vi "Trace Engine.vi"(0 "FPGA VI Reference":refnum<k20>, 7 "Arr Refnum":refnum<vi>, 11 "TraceCluster":refnum<vi>) -> ()   [LabVIEW 2013]
uses:
  <vilib>/rvi/interface/nirviMethod/nirviMethod.xnode
  <vilib>/FPGAPlugInAG/Dynamic/niLvFpga_ReadFifo_Dynamic.vi
  <vilib>/rvi/errors/niLvFpgaMergeErrorWithErrorCode.vi
  Controls/TraceCluster.ctl
  <vilib>/ptbypt/NI_PtbyPt.lvlib
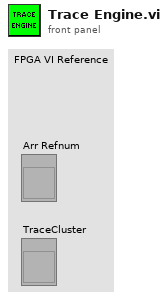
[diagram p1: front panel]
types:
  T1 = typedef "TraceCluster.ctl" = cluster{"PreTriggerPts":i32, "TotalPts":i32, "TriggerLvl":dbl, "PlotStyle":enum16{"Single - Rising Edge", "Single - Falling Edge", "Continuous", "Repeat - Rising Edge", "Repeat - Falling Edge"}, "TriggerChannel":i32, "TraceCtrl":bool}
  T2 = cluster{"rt fifo":refnum<k33>, "FPGA VI Reference":refnum<k20>, "Stored Data":dbl[][], "TraceCluster":T1, "TraceClusterRef":refnum<vi>, "InSync":bool, "Cal Array":dbl[][]}
  T3 = enum16{"Single - Rising Edge", "Single - Falling Edge", "Continuous", "Repeat - Rising Edge", "Repeat - Falling Edge"}
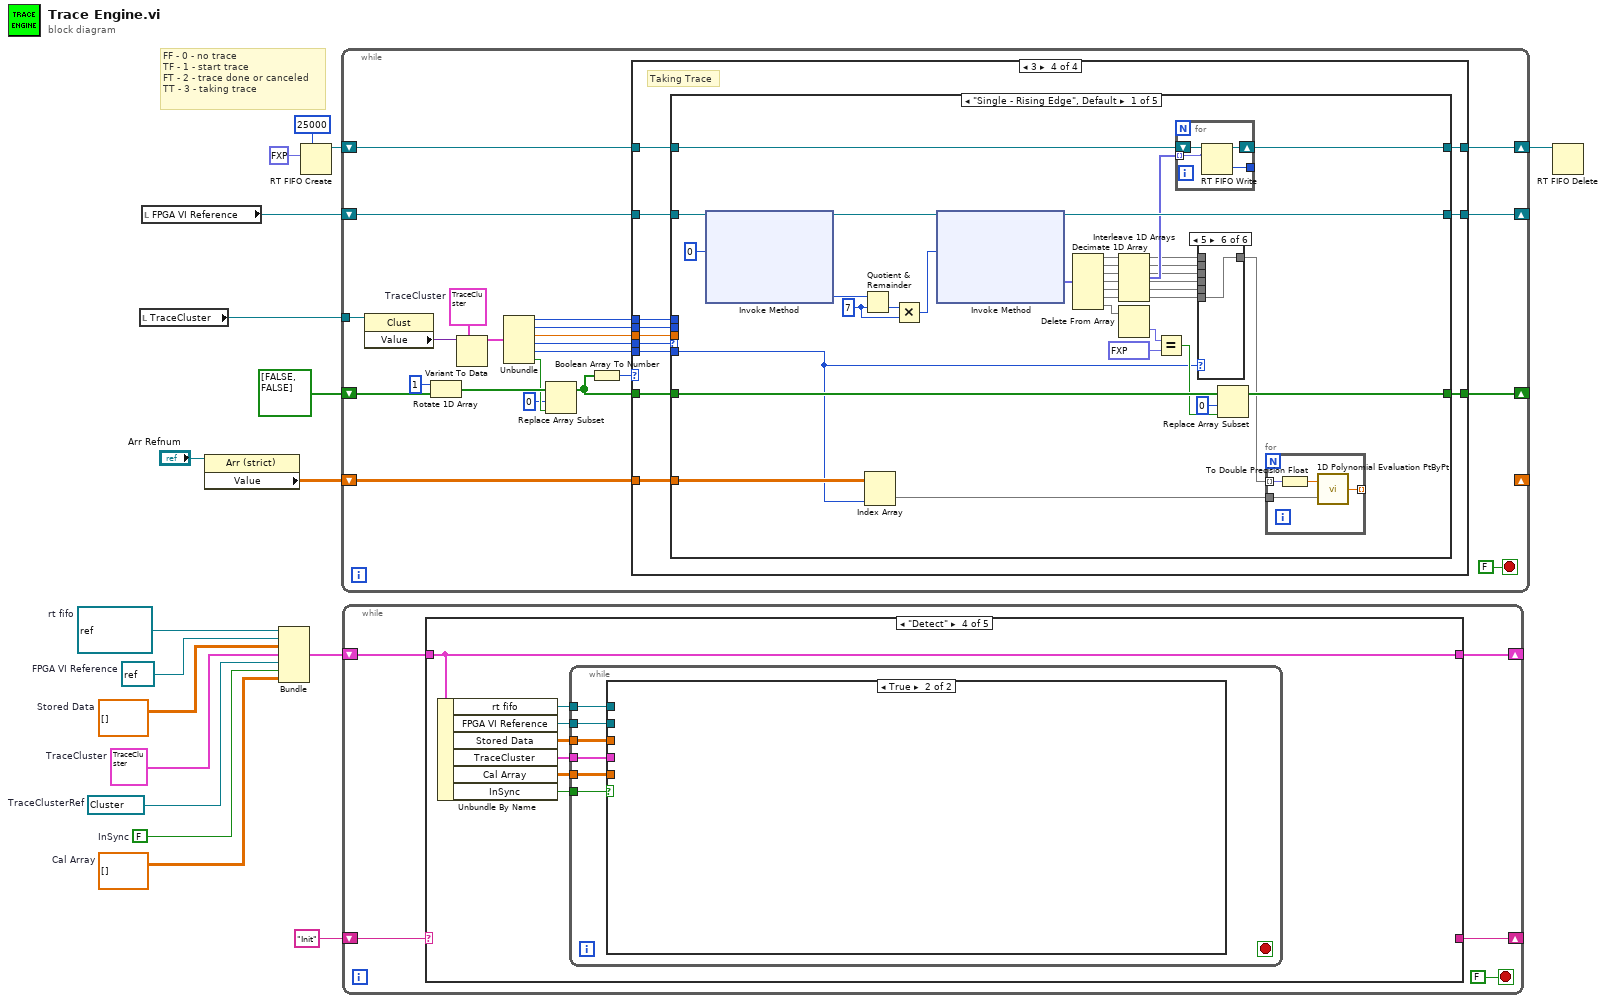
[diagram p0: block diagram]
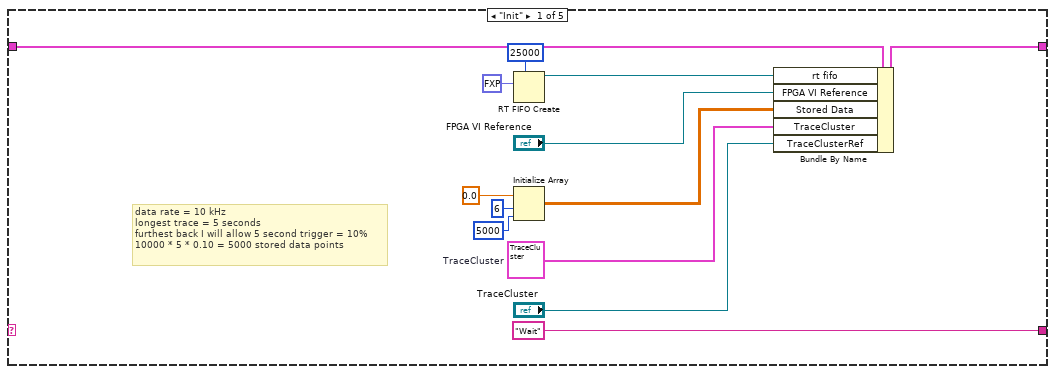
[diagram p2: hidden frame]
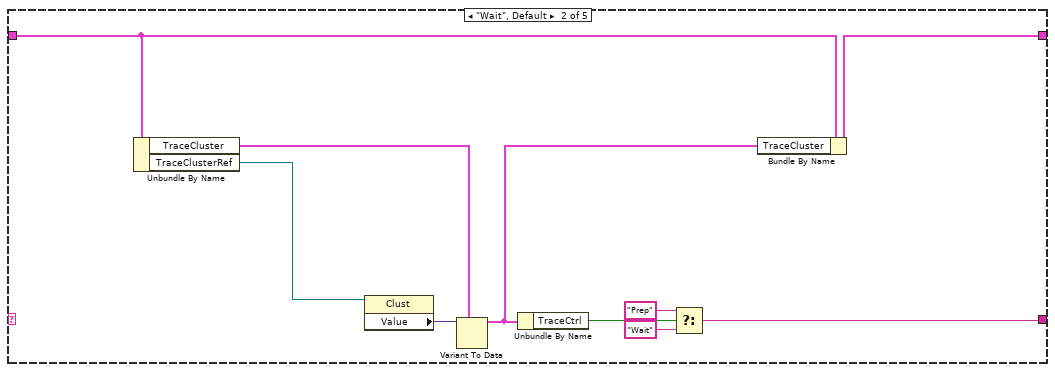
[diagram p3: hidden frame]
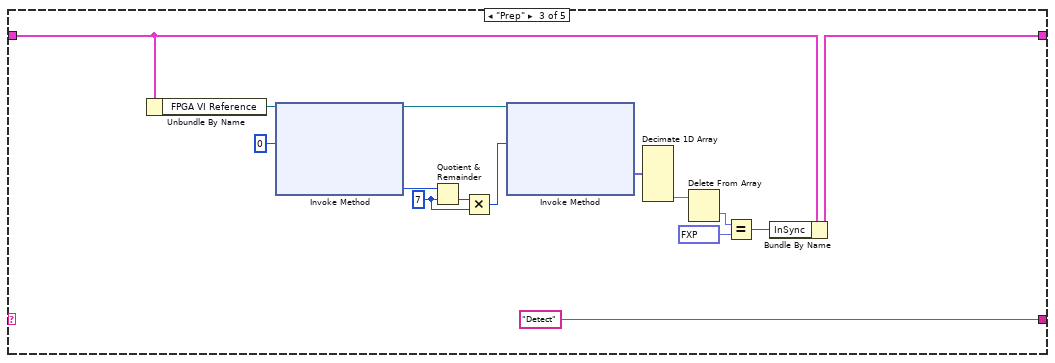
[diagram p4: hidden frame]
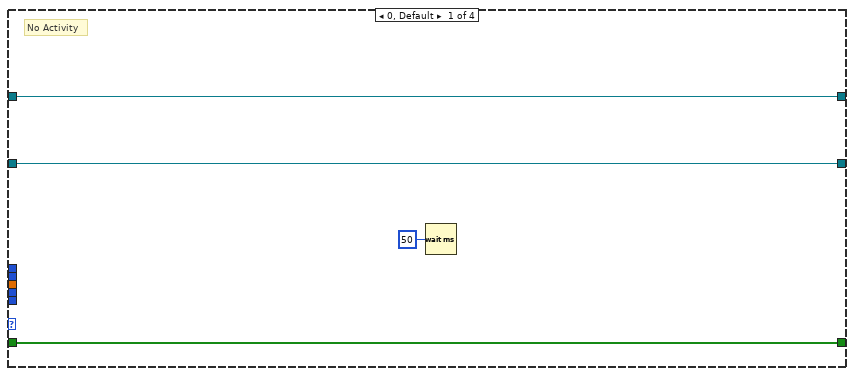
[diagram p7: hidden frame]
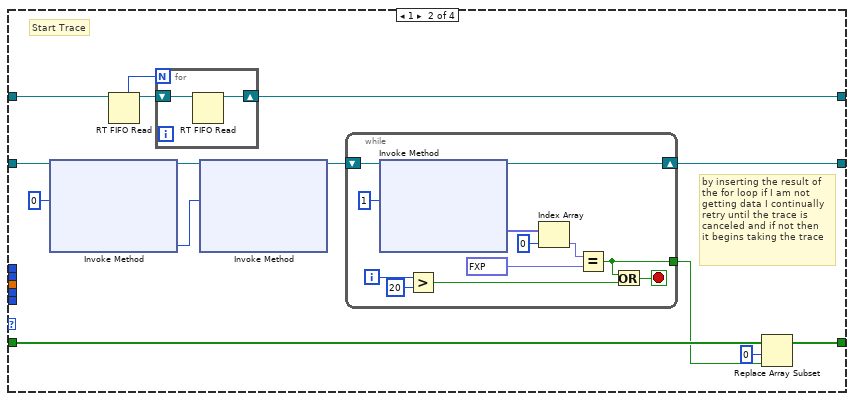
[diagram p8: hidden frame]
diagram:
  w1 = dbl[][] []  # Cal Array
  w3 = FALSE  # InSync
  w4 = refnum<vi> refnum  # TraceClusterRef
  w5 = T1 {"PreTriggerPts"=0, "TotalPts"=0, "TriggerLvl"=0.0, "PlotStyle"=enum."Single - Rising Edge", "TriggerChannel"=0, "TraceCtrl"=FALSE}  # TraceCluster
  w6 = dbl[][] []  # Stored Data
  w7 = refnum<k20> refnum  # FPGA VI Reference
  w8 = refnum<k33> refnum  # rt fifo
  # "FF - 0 - no trace\nTF - 1 - start trace\nFT - 2 - trace done or canceled\nTT - 3 - taking trace"
  n1 = local read "TraceCluster"() -> (w9:refnum<vi>)
  n2 = local read "FPGA VI Reference"() -> (w10:refnum<k20>)
  n3 = property class="Arr (strict)"(reference="Arr Refnum") -> ("Value"=w12:dbl[][])  [unwired: 1 in, 2 out]
  n4 = Bundle("rt fifo"=w8, "FPGA VI Reference"=w7, "Stored Data"=w6, "TraceCluster"=w5, "TraceClusterRef"=w4, "InSync"=w3, "Cal Array"=w1) -> (w2:T2)  [unwired: 1 in]
  n5 = RT FIFO Create(1:fxp<+/-,25,15> 0.0, 4:u32 25000 ("size (10)")) -> (8:w16:refnum<k33>)  [unwired: 6 in, 2 out]
  n6 = while {
    tunnel: w9 -> [w33]
    shift-right: [w22] -> _
    shift-left: bool[] [FALSE, FALSE] -> [w31]
    shift-right: [w24] -> _
    shift-left: w10 -> [w25]
    shift-right: [w20] -> w15
    shift-left: w16 -> [w21]
    shift-right: _ -> [_]
    shift-left: w12 -> [w19]
    stop <- FALSE stop-if-true
    w35 = T1 {"PreTriggerPts"=0, "TotalPts"=0, "TriggerLvl"=0.0, "PlotStyle"=enum."Single - Rising Edge", "TriggerChannel"=0, "TraceCtrl"=FALSE}  # TraceCluster
    n7 = property class="Clust"(reference=w33) -> ("Value"=w34:variant)  [unwired: 1 in, 2 out]
    n8 = Rotate 1D Array(1:w31, 2:1 ("n")) -> (0:w29:bool[])
    n9 = Variant To Data(type=w35, Variant=w34) -> (data=w32:T1)  [unwired: 1 in, 1 out]
    n10 = Unbundle(w32) -> ("PreTriggerPts"=w36:i32, "TotalPts"=w37:i32, "TriggerLvl"=w38:dbl, "PlotStyle"=w40:T3, "TriggerChannel"=w39:i32, "TraceCtrl"=w28:bool)
    n11 = Replace Array Subset(array=w29, new element=w28, index=0) -> (w23:bool[])
    n12 = Boolean Array To Number(Boolean array=w23) -> (number=w26:u32)
    n13 = case shown="3" w26 {
      tunnel: w25 -> [w44 w59 w76 w88]
      tunnel: w40 -> [_ _ _ w84]
      tunnel: w39 -> [_ _ _ w83]
      tunnel: w38 -> [_ _ _ w85]
      tunnel: w37 -> [_ _ _ w86]
      tunnel: w36 -> [_ _ _ w87]
      tunnel: [w44 w54 w76 w80] -> w24
      tunnel: w23 -> [w43 w53 w75 w79]
      tunnel: [w43 w52 w75 w78] -> w22
      tunnel: w21 -> [w42 w49 w74 w82]
      tunnel: [w42 w46 w74 w81] -> w20
      tunnel: w19 -> [_ _ _ w77]
      frame 0, Default {
        # "No Activity"
        n14 = Wait (ms)(milliseconds to wait=u32 50) -> ()  [unwired: 1 out]
      }
      frame 1 {
        # "Start Trace"
        # "by inserting the result of\nthe for loop if I am not\ngetting data I continually\nretry until the trace is\ncanceled and if not then\nit begins taking the trace"
        n15 = xnode "Invoke Method"("FPGA VI Reference In"=w59, "Number of Elements"=u32 0) -> ("FPGA VI Reference Out"=w58:refnum<k20>, "Elements Remaining"=w55:u32)  [unwired: 2 in, 2 out]
        n16 = RT FIFO Read(0:w49) -> (7:w47:u32, 8:w48:refnum<k33>)  [unwired: 3 in, 3 out]
        n17 = for {
          N: w47 -> [_]
          shift-right: [w60] -> w46
          shift-left: w48 -> [w61]
          n18 = RT FIFO Read(0:w61) -> (8:w60:refnum<k33>)  [unwired: 3 in, 4 out]
        }
        n19 = xnode "Invoke Method"("FPGA VI Reference In"=w58, "Number of Elements"=w55) -> ("FPGA VI Reference Out"=w57:refnum<k20>)  [unwired: 2 in, 3 out]
        n20 = while {
          shift-right: [w64] -> w54
          shift-left: w57 -> [w72]
          tunnel: [w62] -> w50
          i -> [w67]
          stop <- w65 stop-if-true
          n21 = xnode "Invoke Method"("FPGA VI Reference In"=w72, "Number of Elements"=u32 1) -> ("FPGA VI Reference Out"=w64:refnum<k20>, "Data"=w70:fxp<+/-,25,15>[])  [unwired: 2 in, 2 out]
          n22 = Greater?(x=w67, y=20) -> (0:w63:bool)
          n23 = Index Array(array=w70, index=0) -> (element=w68:fxp<+/-,25,15>)
          n24 = Equal?(x=w68, y=fxp<+/-,1,15> -16384.0) -> (x = y?=w62:bool)
          n25 = Or(x=w62, y=w63) -> (x .or. y?=w65:bool)
        }
        n26 = Replace Array Subset(array=w53, new element=w50, index=0) -> (w52:bool[])
      }
      frame 2 {
        # "Trace Canceled OR Trace Complete"
      }
      frame 3 {
        # "Taking Trace"
        n27 = case shown="\"Single - Rising Edge\", Default" w84 {
          tunnel: w83 -> [w96 _ _ _ _]
          tunnel: w85 -> [_ _ _ _ _]
          tunnel: w86 -> [_ _ _ _ _]
          tunnel: w87 -> [_ _ _ _ _]
          tunnel: w88 -> [w116 _ _ _ _]
          tunnel: w82 -> [w114 _ _ _ _]
          tunnel: [w109 _ _ _ _] -> w81
          tunnel: [w108 _ _ _ _] -> w80
          tunnel: w79 -> [w104 _ _ _ _]
          tunnel: [w103 _ _ _ _] -> w78
          tunnel: w77 -> [w98 _ _ _ _]
          frame "Single - Rising Edge", Default {
            w111 = u32 7 ("y")
            n28 = xnode "Invoke Method"("FPGA VI Reference In"=w116, "Number of Elements"=u32 0) -> ("FPGA VI Reference Out"=w115:refnum<k20>, "Elements Remaining"=w113:u32)  [unwired: 2 in, 2 out]
            n29 = Quotient & Remainder(x=w113, y=w111) -> (floor(x/y)=w112:u32)  [unwired: 1 out]
            n30 = Index Array(array=w98, index (col)=w96) -> (element=w97:dbl[])  [unwired: 1 in]
            n31 = Multiply(x=w112, y=w111) -> (x*y=w110:u32)
            n32 = xnode "Invoke Method"("FPGA VI Reference In"=w115, "Number of Elements"=w110) -> ("FPGA VI Reference Out"=w108:refnum<k20>, "Data"=w107:fxp<+/-,25,15>[])  [unwired: 2 in, 2 out]
            n33 = Decimate 1D Array(w107) -> (w95:fxp<+/-,25,15>[], w94:fxp<+/-,25,15>[], w93:fxp<+/-,25,15>[], w92:fxp<+/-,25,15>[], w91:fxp<+/-,25,15>[], w90:fxp<+/-,25,15>[], w100:fxp<+/-,25,15>[])
            n34 = Interleave 1D Arrays(w95, w94, w93, w92, w91, w90) -> (w99:fxp<+/-,25,15>[])
            n35 = Delete From Array(array=w100) -> (deleted portion=w106:fxp<+/-,25,15>)  [unwired: 2 in, 1 out]
            n36 = Equal?(x=w106, y=fxp<+/-,25,15> -16384.0) -> (x = y?=w102:bool)
            n37 = for {
              tunnel: [w128] -> _ mode=indexing
              shift-right: [w130] -> w109
              shift-left: w114 -> [w131]
              tunnel: [w129] -> _
              tunnel: w99 -> [w128] mode=indexing
              n38 = RT FIFO Write(0:w131, 1:w128) -> (7:w129:u32, 8:w130:refnum<k33>)  [unwired: 3 in, 2 out]
            }
            n39 = case shown="5" w96 {
              tunnel: w95 -> [w118 _ _ _ _ _]
              tunnel: w94 -> [_ w119 _ _ _ _]
              tunnel: w93 -> [_ _ w120 _ _ _]
              tunnel: w92 -> [_ _ _ w121 _ _]
              tunnel: w91 -> [_ _ _ _ w122 _]
              tunnel: w90 -> [_ _ _ _ _ w123]
              tunnel: [w118 w119 w120 w121 w122 w123] -> w89
              frame 0, Default {
              }
              frame 1 {
              }
              frame 2 {
              }
              frame 3 {
              }
              frame 4 {
              }
              frame 5 {
              }
            }
            n40 = Replace Array Subset(array=w104, new element=w102, index=0) -> (w103:bool[])
            n41 = for {
              tunnel: w97 -> [w127]
              tunnel: w89 -> [w125] mode=indexing
              tunnel: [w126] -> _ mode=indexing
              n42 = To Double Precision Float(number=w125) -> (double precision float=w124:dbl)
              n43 = call <vilib>:"1D Polynomial Evaluation PtByPt.vi"("Coefficients: a"=w127, "x"=w124) -> ("y"=w126:dbl)
            }
          }
          frame "Single - Falling Edge" {
          }
          frame "Continuous" {
          }
          frame "Repeat - Rising Edge" {
          }
          frame "Repeat - Falling Edge" {
          }
        }
      }
    }
  }
  n44 = while {
    shift-right: [w134] -> _
    shift-left: "Init" -> [w135]
    shift-right: [w132] -> _
    shift-left: w2 -> [w133]
    stop <- FALSE stop-if-true
    n45 = case shown="\"Detect\"" w135 {
      tunnel: ["Wait" w155 "Detect" _ _] -> w134
      tunnel: w133 -> [w143 w152 w162 w181 _]
      tunnel: [w137 w151 w161 w181 _] -> w132
      frame "Init" {
        w139 = T1 {"PreTriggerPts"=0, "TotalPts"=0, "TriggerLvl"=0.0, "PlotStyle"=enum."Single - Rising Edge", "TriggerChannel"=0, "TraceCtrl"=FALSE}  # TraceCluster
        # "data rate = 10 kHz\nlongest trace = 5 seconds\nfurthest back I will allow 5 second trigger = 10%\n10000 * 5 * 0.10 = 5000 stored data points"
        n46 = RT FIFO Create(1:fxp<+/-,25,15> 0.0, 4:u32 25000 ("size (10)")) -> (8:w142:refnum<k33>)  [unwired: 6 in, 2 out]
        n47 = Initialize Array(0.0 ("element"), 6 ("dimension size"), 5000 ("dimension size")) -> (w140:dbl[][])
        n48 = Bundle By Name(cluster=w143, "rt fifo"=w142, "FPGA VI Reference"="FPGA VI Reference", "Stored Data"=w140, "TraceCluster"=w139, "TraceClusterRef"="TraceCluster") -> (w137:T2)
      }
      frame "Wait", Default {
        n49 = Unbundle By Name(w152) -> ("TraceCluster"=w153:T1, "TraceClusterRef"=w154:refnum<vi>)
        n50 = property class="Clust"(reference=w154) -> ("Value"=w159:variant)  [unwired: 1 in, 2 out]
        n51 = Variant To Data(type=w153, Variant=w159) -> (data=w150:T1)  [unwired: 1 in, 1 out]
        n52 = Unbundle By Name(w150) -> ("TraceCtrl"=w158:bool)
        n53 = Select(t="Prep", s=w158, f="Wait") -> (s? t:f=w155:string)
        n54 = Bundle By Name(cluster=w152, "TraceCluster"=w150) -> (w151:T2)
      }
      frame "Prep" {
        w168 = u32 7 ("y")
        n55 = Unbundle By Name(w162) -> ("FPGA VI Reference"=w164:refnum<k20>)
        n56 = xnode "Invoke Method"("FPGA VI Reference In"=w164, "Number of Elements"=u32 0) -> ("FPGA VI Reference Out"=w163:refnum<k20>, "Elements Remaining"=w166:u32)  [unwired: 2 in, 2 out]
        n57 = Quotient & Remainder(x=w166, y=w168) -> (floor(x/y)=w167:u32)  [unwired: 1 out]
        n58 = Multiply(x=w167, y=w168) -> (x*y=w169:u32)
        n59 = xnode "Invoke Method"("FPGA VI Reference In"=w163, "Number of Elements"=w169) -> ("Data"=w170:fxp<+/-,25,15>[])  [unwired: 2 in, 3 out]
        n60 = Decimate 1D Array(w170) -> (w173:fxp<+/-,25,15>[])  [unwired: 6 out]
        n61 = Delete From Array(array=w173) -> (deleted portion=w171:fxp<+/-,25,15>)  [unwired: 2 in, 1 out]
        n62 = Equal?(x=w171, y=fxp<+/-,25,15> -16384.0) -> (x = y?=w160:bool)
        n63 = Bundle By Name(cluster=w162, "InSync"=w160) -> (w161:T2)
      }
      frame "Detect" {
        n64 = Unbundle By Name(w181) -> ("rt fifo"=w175:refnum<k33>, "FPGA VI Reference"=w176:refnum<k20>, "Stored Data"=w177:dbl[][], "TraceCluster"=w178:T1, "Cal Array"=w179:dbl[][], "InSync"=w180:bool)
        n65 = while {
          tunnel: w180 -> [w187]
          tunnel: w179 -> [w186]
          tunnel: w178 -> [w185]
          tunnel: w177 -> [w184]
          tunnel: w176 -> [w183]
          tunnel: w175 -> [w182]
          stop <- _ stop-if-true
          n66 = case shown="True" w187 {
            tunnel: w186 -> [_ _]
            tunnel: w185 -> [_ _]
            tunnel: w184 -> [_ _]
            tunnel: w183 -> [_ _]
            tunnel: w182 -> [_ _]
            frame False {
            }
            frame True {
            }
          }
        }
      }
      frame "Send" {
      }
    }
  }
  n67 = RT FIFO Delete(0:w15) -> ()  [unwired: 2 in, 1 out]
